vi "Load Configuration Settings from XML.vi"(8 "error in (no error)":errorcluster caption="错误输入（无错误）", 11 "用户配置输入":T1) -> (0 "error out":errorcluster caption="错误输出", 3 "用户配置输出":T1)   [LabVIEW 2022 SP3]
uses:
  controls/User Specified Data_self.ctl
  controls/HW Configuration_self.ctl
  controls/Simulated Signal Type_self.ctl
  controls/Analysis Configuration_self.ctl
  controls/New Data Behavior_self.ctl
  <vilib>/Utility/xml.llb/Read From XML File(string).vi
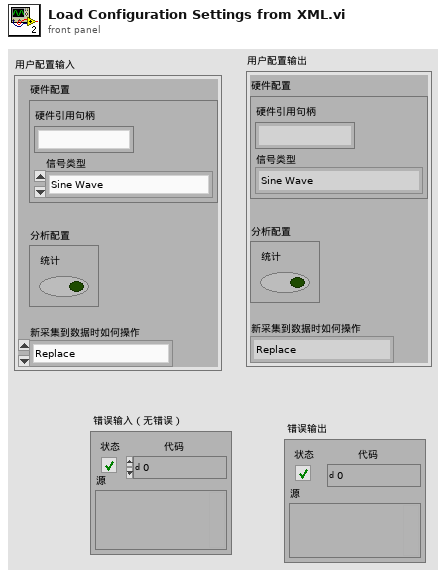
[diagram p1: front panel]
types:
  T1 = typedef "User Specified Data_self.ctl" = cluster{"硬件配置":T2, "分析配置":T4, "新采集到数据时如何操作":T5}
  T2 = typedef "HW Configuration_self.ctl" = cluster{"硬件引用句柄":string, "信号类型":T3}
  T3 = typedef "Simulated Signal Type_self.ctl" = enum16{"Sine Wave", "Square Wave"}
  T4 = typedef "Analysis Configuration_self.ctl" = cluster{"统计":bool}
  T5 = typedef "New Data Behavior_self.ctl" = enum16{"Replace", "Overlay", "Append"}
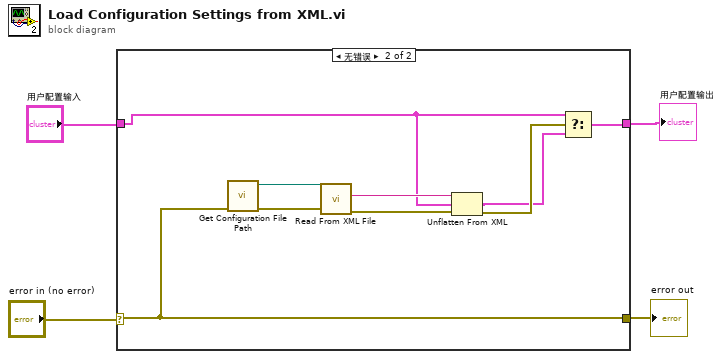
[diagram p0: block diagram]
diagram:
  n1 = case shown="无错误" "error in (no error)" {
    selector: "error in (no error)" -> [w6 w15]
    tunnel: [w6 w15] -> w3
    tunnel: "用户配置输入" -> [w5 w7]
    tunnel: [w5 w9] -> w2
    frame Error {
    }
    frame No Error {
      n2 = call "Get Configuration File Path.vi"("error in (no error)"=w15) -> ("error out"=w14:errorcluster, "XML 文件路径"=w13:path)  [unwired: 9 in]
      n3 = call-poly <vilib>:"Read From XML File.vi"("error in (no error)"=w14, "XML File Path"=w13) -> ("error out"=w12:errorcluster, "XML Elements"=w11:string)  [unwired: 7 in, 1 out]
      n4 = Unflatten From XML(xml string=w11, type=w7, error in (no error)=w12) -> (value=w8:T1, error out=w10:errorcluster)
      n5 = Select(t=w7, s=w10, f=w8) -> (s? t:f=w9:T1)
    }
  }
  "error out" <- w3
  "用户配置输出" <- w2
